vi "Test Speaker Switching.vi"() -> ()   [LabVIEW 2012]
uses:
  Reusable/Switch/Switch.lvclass
panel:
  in  "Filter":bool=TRUE
  out "Time since Switch":dbl
  out "current time":timestamp format="%<%H:%M:%S%2u>T"
  out "Last Switch":timestamp format="%<%H:%M:%S%2u>T"
  in  "Speaker":bool=TRUE
  in  "Flags":T1
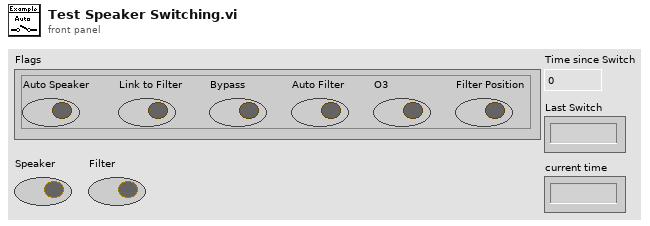
[diagram p1: front panel]
types:
  T1 = cluster{"Auto Speaker":bool, "Link to Filter":bool, "Bypass":bool, "Auto Filter":bool, "O3":bool, "Filter Position":bool}
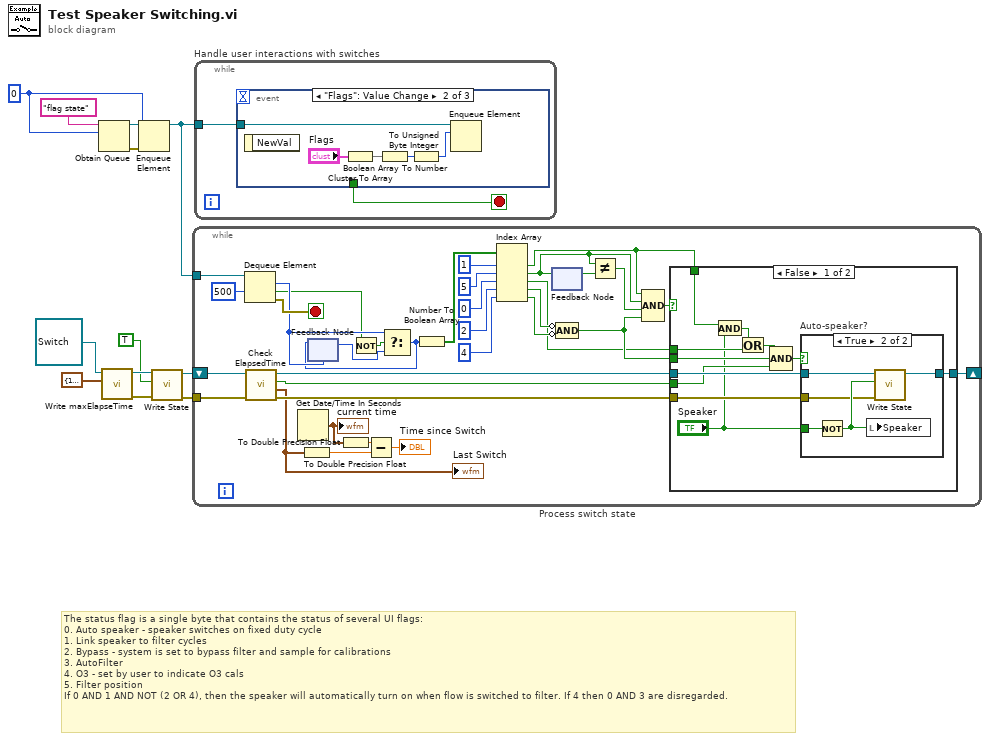
[diagram p0: block diagram]
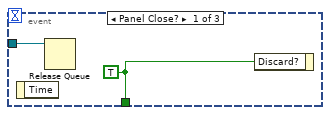
[diagram p2: hidden frame]
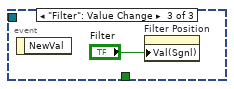
[diagram p3: hidden frame]
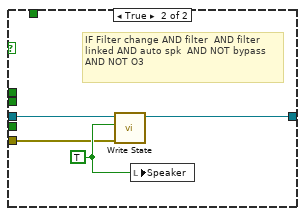
[diagram p5: hidden frame]
diagram:
  w7 = u8 0
  # "The status flag is a single byte that contains the status of several UI flags: \n0. Auto speaker - speaker switches on fixed duty cycle \n1. Link speaker to filter cycles \n2. Bypass - system is set to bypass filter and sample for calibrations \n3. AutoFilter \n4. O3 - set by user to indicate O3 cals \n5. Filter position \nIf 0 AND 1 AND NOT (2 OR 4), then the speaker will automatically turn on when flow is switched to filter. If 4 then 0 AND 3 are disregarded."
  n1 = Obtain Queue(name (unnamed)="flag state", element data type=w7) -> (queue out=w10:refnum<queue>, error out=w9:errorcluster)  [unwired: 3 in, 1 out]
  n2 = call "Write maxElapseTime.vi"("maxElapsedTime"=cluster{"true":dbl, "false":dbl} {"true"=10.0, "false"=5.0}, "Switch in"=refnum<class "Switch.lvclass"> refnum ("Switch.lvclass")) -> ("error out"=w5:errorcluster, "Switch out"=w6:refnum<class "Switch.lvclass">)  [unwired: 8 in]
  n3 = Enqueue Element(queue=w10, element=w7, error in (no error)=w9) -> (queue out=w8:refnum<queue>)  [unwired: 1 in, 2 out]
  n4 = call-dynamic "Write State.vi"("error in"=w5, "State"=TRUE, "Switch in"=w6) -> ("error out"=w2:errorcluster, "Switch out"=w3:refnum<class "Switch.lvclass">)  [unwired: 7 in]
  n5 = while "Process switch state" {
    tunnel: w8 -> [w46]
    tunnel: w2 -> [w28]
    shift-right: [w25] -> _
    shift-left: w3 -> [w29]
    stop <- w45 stop-if-true
    n6 = Dequeue Element(queue=w46, timeout in ms (-1)=500) -> (element=w42:u8, timed out?=w41:bool, error out=w45:errorcluster)  [unwired: 1 in, 1 out]
    n7 = call-dynamic "Check ElapsedTime.vi"("error in"=w28, "Switch in"=w29) -> ("error out"=w27:errorcluster, "LastSwitch"=w15:timestamp, "TimeElapsed?"=w21:bool, "Switch out"=w26:refnum<class "Switch.lvclass">)  [unwired: 6 in]
    "Last Switch" <- w15
    n8 = Get Date/Time In Seconds() -> (seconds since 1Jan1904=w16:timestamp)
    "current time" <- w16
    n9 = To Double Precision Float(number=w15) -> (double precision float=w14:dbl)
    n10 = feedback #1(w42) -> (w43:u8)
    n11 = To Double Precision Float(number=w16) -> (double precision float=w13:dbl)
    n12 = Not(x=w41) -> (.not. x?=w44:bool)
    n13 = Subtract(x=w13, y=w14) -> (x-y=→"Time since Switch":dbl)
    n14 = Select(t=w42, s=w44, f=w43) -> (s? t:f=w22:u8)
    n15 = feedback-in #1(w22) -> ()
    n16 = Number To Boolean Array(number=w22) -> (Boolean array=w39:bool[])
    n17 = Index Array(array=w39, index #1=1 ("index"), index #2=5 ("index"), index #3=0 ("index"), index #4=2 ("index"), index #5=4 ("index")) -> (element #1=w18:bool, element #2=w17:bool, element #3=w19:bool, element #4=w32:bool, element #5=w31:bool)
    n18 = feedback #2() -> (w37:bool)  [unwired: 1 in]
    n19 = feedback-in #2(w17) -> ()
    n20 = Compound Arithmetic op=AND(invert w32, invert w31) -> (w20:bool)
    n21 = Not Equal?(x=w17, y=w37) -> (x != y?=w40:bool)
    n22 = Compound Arithmetic op=AND(w18, w17, w40, w20) -> (w30:bool)
    n23 = case shown="False" w30 {
      tunnel: w27 -> [w57 w64]
      tunnel: w26 -> [w56 w66]
      tunnel: [w55 w65] -> w25
      tunnel: w21 -> [w54 _]
      tunnel: w20 -> [w53 _]
      tunnel: w19 -> [w49 _]
      tunnel: w18 -> [w51 _]
      frame False {
        n24 = And(x=w51, y="Speaker") -> (x .and. y?=w50:bool)
        n25 = Or(x=w50, y=w49) -> (x .or. y?=w48:bool)
        n26 = Compound Arithmetic op=AND(w48, w53, w54) -> (w52:bool)
        n27 = case "Auto-speaker?" shown="True" w52 {
          tunnel: w57 -> [_ w60]
          tunnel: w56 -> [w58 w62]
          tunnel: [w58 w61] -> w55
          tunnel: "Speaker" -> [_ w59]
          frame False {
            # "O3 OR bypass == TRUE"
          }
          frame True {
            n28 = Not(x=w59) -> (.not. x?=w63:bool)
            n29 = local write "Speaker"(w63) -> ()
            n30 = call-dynamic "Write State.vi"("error in"=w60, "State"=w63, "Switch in"=w62) -> ("Switch out"=w61:refnum<class "Switch.lvclass">)  [unwired: 7 in, 1 out]
          }
        }
      }
      frame True {
        w67 = TRUE ("drive")
        # "IF Filter change AND filter  AND filter linked AND auto spk  AND NOT bypass  AND NOT O3"
        n31 = call-dynamic "Write State.vi"("error in"=w64, "State"=w67, "Switch in"=w66) -> ("Switch out"=w65:refnum<class "Switch.lvclass">)  [unwired: 7 in, 1 out]
        n32 = local write "Speaker"(w67) -> ()
      }
    }
  }
  n33 = while "Handle user interactions with switches" {
    tunnel: w8 -> [w68]
    stop <- w69 stop-if-true
    n34 = event shown="[1] \"Flags\": Value Change" {
      selector: _ -> [_ _ _]
      dyn-events: _ -> [_ _ _]
      timeout: _ -> [_ _ _]
      tunnel: [w71 _ _] -> w69
      tunnel: w68 -> [w70 w76 _]
      event Panel Close? {
        w71 = TRUE
        n35 = event-data() -> ()  [unwired: 1 in, 1 out]
        n36 = Release Queue(queue=w70) -> ()  [unwired: 2 in, 3 out]
        n37 = event-data("Discard?"=w71) -> ()  [unwired: 1 in, 1 out]
      }
      event "Flags": Value Change {
        n38 = event-data() -> ()  [unwired: 1 in, 1 out]
        n39 = Cluster To Array(cluster="Flags") -> (array=w74:bool[])
        n40 = Boolean Array To Number(Boolean array=w74) -> (number=w73:u32)
        n41 = To Unsigned Byte Integer(number=w73) -> (unsigned 8bit integer=w72:u8)
        n42 = Enqueue Element(queue=w76, element=w72) -> ()  [unwired: 2 in, 3 out]
      }
      event "Filter": Value Change {
        n43 = event-data() -> ()  [unwired: 1 in, 1 out]
        n44 = property on="Filter Position" class="Bool (strict)"("Val(Sgnl)"="Filter") -> ()  [unwired: 2 in, 2 out]
      }
    }
  }
